vi "RSNRPZ Set Scope Measurement Equivalent Sampling.vi"(8 "error in (no error)":errorcluster, 9 "Scope Meas Equiv Sampling (On)":bool=TRUE, 10 "Channel (1)":i32=1, 11 "VISA session":refnum<visa-resource-name> caption="VISA resource name") -> (0 "error out":errorcluster, 3 "dup VISA session":refnum<visa-resource-name> caption="VISA resource name")   [LabVIEW 2010]
doc: "This VI activates or deactivates the automatic equivalent sampling mode during automatic pulse analysis.\nIf equivalent sampling is enabled, the sensor tries to measure the time parameters (mainly rise/fall times) of the pulse with a high resolution by doing equivalent sampling.\nTo do the equivalent sampling a periodic signal is mandatory. The sensor decides automatically if equivalent sampling is possible. To get the resolution of the measured time parameter the VI \"RSNRPZ Get Scope Measurement Sample Period.vi\" could be used.\n\nNote:\n1) This VI is only available for NRP-Z81.\n\nRemote-control command(s):\nSENS:TRAC:MEAS:TRANS:ESAM:AUTO"
uses:
  rsnrpz_32.dll
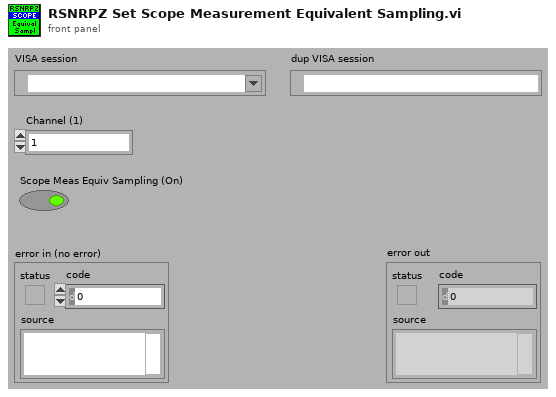
[diagram p1: front panel]
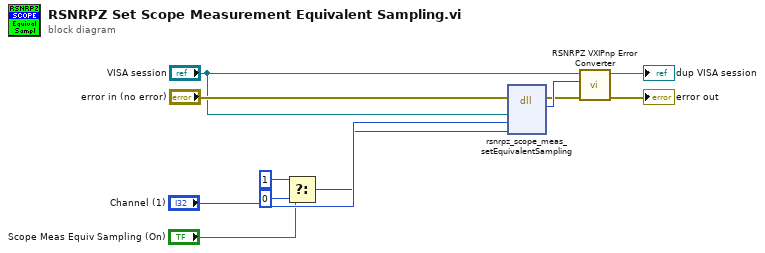
[diagram p0: block diagram]
diagram:
  n1 = Select(t=i16 1, s="Scope Meas Equiv Sampling (On)", f=i16 0) -> (s? t:f=w7:i16)
  n2 = dll-call lib="rsnrpz_32.dll" fn="rsnrpz_scope_meas_setEquivalentSampling"(error in="error in (no error)", "Instrument Handle"="VISA session", "Channel"="Channel (1)", "Scope Meas Equiv Sampling"=w7) -> (error out=w5:errorcluster, w6:i32)  [unwired: 5 in, 1 out]
  n3 = call <instrlib>:"RSNRPZ VXIPnp Error Converter.vi"("error in"=w5, "VXIPnp error code"=w6, "VISA session"="VISA session") -> ("error out"=→"error out":errorcluster, "dup VISA session"=→"dup VISA session":refnum<visa-resource-name>)  [unwired: 7 in]
